vi "uart data_main — kopia.vi"() -> ()   [LabVIEW 2015]
uses:
  data_typedef.ctl
  C:/Users/Arkadiusz/SkyDrive/Dokumenty/NordicSemiconductor/LabVIEW/UART_Accelero/uart data_akcelerometr/NordicDatabaseDLL.dll
  NordicDatabaseDLL.dll
  <vilib>/Instr/_visa.llb/VISA Configure Serial Port (Instr).vi
panel:
  out "Accelero Chart":T1(graph)
  out "Temperature Chart":dbl[](graph)
  in  "stop":bool
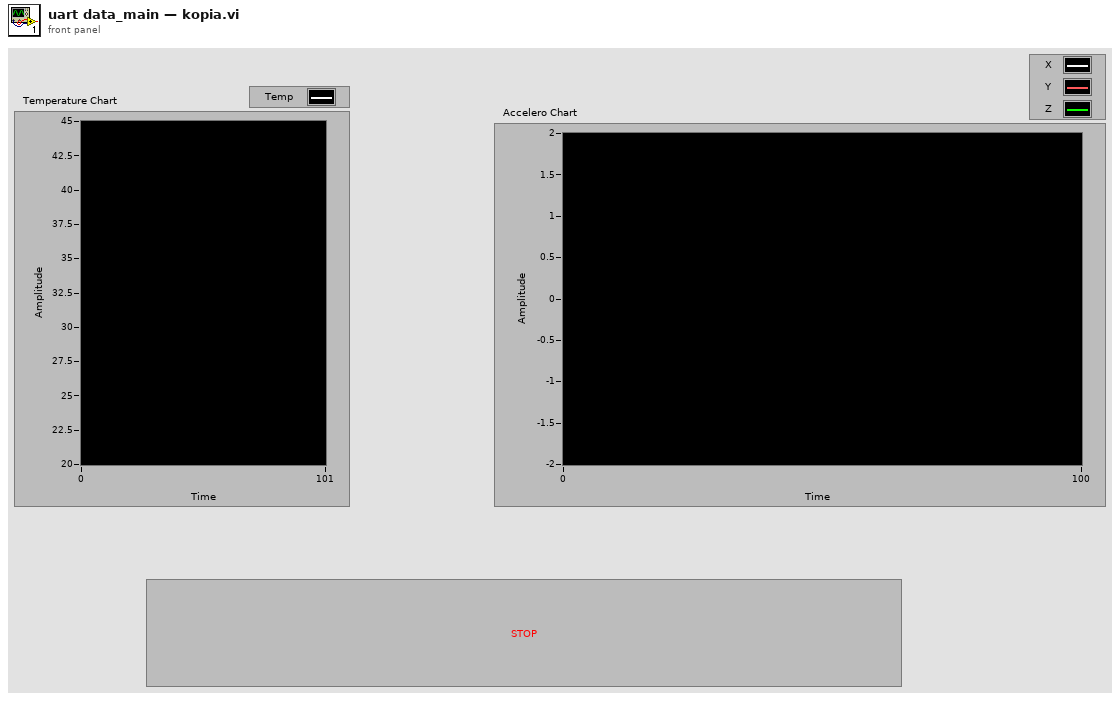
[diagram p1: front panel]
types:
  T1 = cluster{"X element out":dbl, "X element out":dbl, "Z element out":dbl}
  T2 = cluster{"Z element out":dbl, "X element out":dbl, "X element out 2":dbl}[]
  T3 = typedef "data_typedef.ctl" = cluster{"Accelero Array":dbl[], "Z out":dbl[], "Y out":dbl[], "X out":dbl[], "Numeric":i32}
  T4 = typedef "DBEnum.ctl" = enum16{"Temperature", "HeartRate", "XAccelero", "YAccelero", "ZAccelero"}
  T5 = cluster{"X element out":dbl, "Y element out":dbl, "Z element out":dbl}
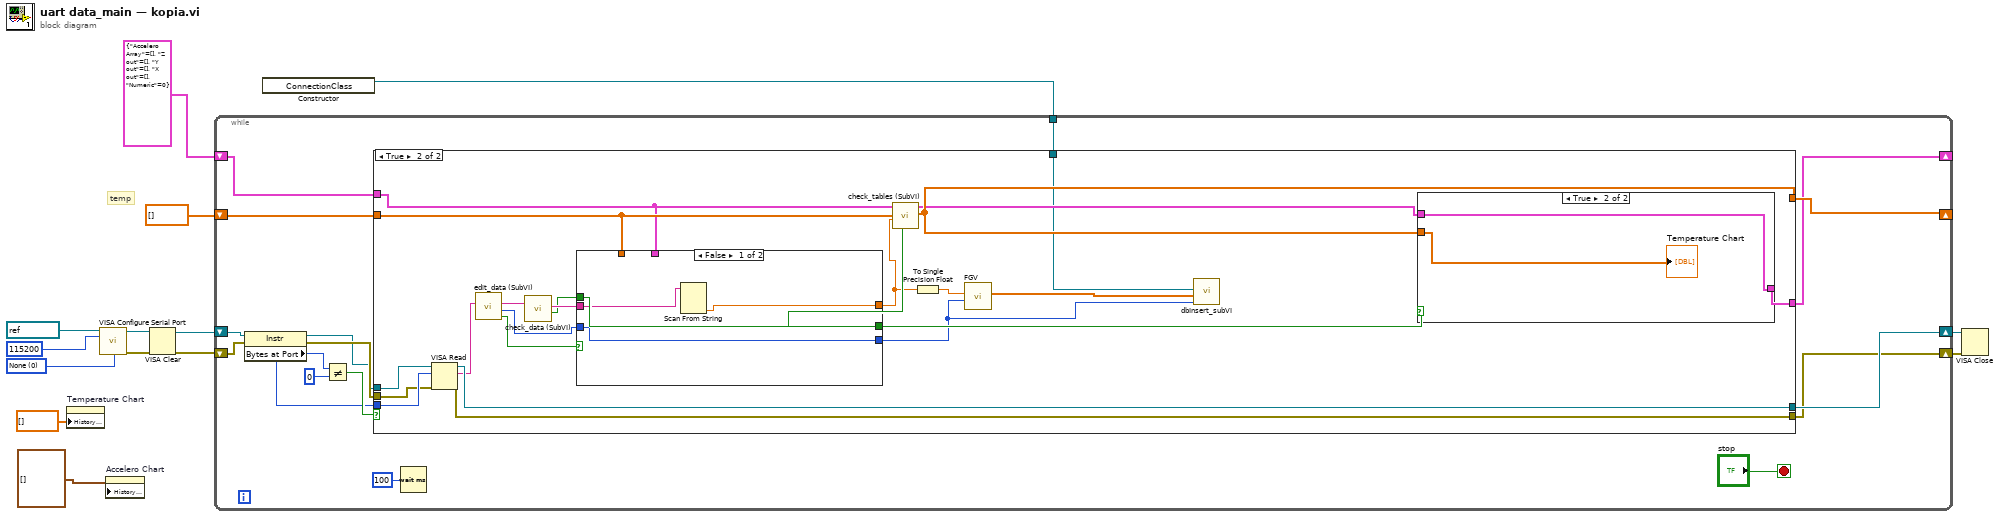
[diagram p0: block diagram]
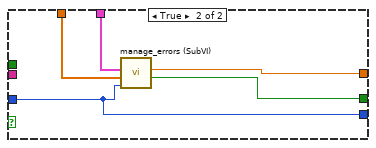
[diagram p3: hidden frame]
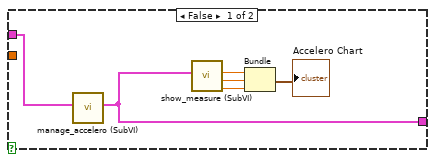
[diagram p4: hidden frame]
diagram:
  w10 = u16 0 items=["None", "XON/XOFF", "RTS/CTS", "XON/XOFF & RTS/CTS", "DTR/DSR", "XON/XOFF & DTR/DSR"] ("flow control (0:none)")
  # "temp"
  n1 = property on="Temperature Chart" class="WFChart (strict)"("History Data"=dbl[] []) -> ()  [unwired: 2 in, 2 out]
  n2 = call-poly "VISA Configure Serial Port"("VISA resource name"=refnum<visa-resource-name> "COM5", "baud rate (9600)"=u32 115200, "flow control (0:none)"=w10) -> ("VISA resource name out"=w6:refnum<visa-resource-name>, "error out"=w5:errorcluster)  [unwired: 11 in]
  n3 = property on="Accelero Chart" class="WFChart (strict)"("History Data"=T2 []) -> ()  [unwired: 2 in, 2 out]
  n4 = VISA Clear(VISA resource name=w6, error in (no error)=w5) -> (VISA resource name out=w7:refnum<visa-resource-name>, error out=w8:errorcluster)
  n5 = constructor class="ConnectionClass"() -> (reference out=w1:refnum<k24>)  [unwired: 3 in, 2 out]
  n6 = while {
    shift-right: [w29] -> w12
    shift-left: w7 -> [w28]
    shift-right: [w25] -> w11
    shift-left: w8 -> [w26]
    shift-right: [w18] -> _
    shift-left: dbl[] [] -> [w21]
    shift-right: [w16] -> _
    shift-left: T3 {"Accelero Array"=[], "Z out"=[], "Y out"=[], "X out"=[], "Numeric"=0} ("Tabs") -> [w17]
    tunnel: w1 -> [w15]
    stop <- "stop" stop-if-true
    # "main loop"
    n7 = property class="Instr"(reference=w28, error in=w26) -> (reference out=w24:refnum<visa-resource-name>, error out=w27:errorcluster, "Bytes at Port"=w20:u32)
    n8 = Not Equal?(x=w20, y=u32 0) -> (x != y?=w22:bool)
    n9 = case shown="True" w22 {
      tunnel: [w34 w56] -> w29
      tunnel: w20 -> [_ w55]
      tunnel: w27 -> [w33 w54]
      tunnel: [w33 w53] -> w25
      tunnel: w24 -> [w34 w52]
      tunnel: w21 -> [w32 w46]
      tunnel: [w32 w50] -> w18
      tunnel: w17 -> [w31 w44]
      tunnel: [w31 w49] -> w16
      tunnel: w15 -> [_ w36]
      frame False {
      }
      frame True {
        # "true"
        n10 = VISA Read(VISA resource name=w52, byte count=w55, error in (no error)=w54) -> (VISA resource name out=w56:refnum<visa-resource-name>, read buffer=w41:string, error out=w53:errorcluster)  [unwired: 1 out]
        n11 = call "edit_data (SubVI).vi"("data in"=w41) -> ("error bool out"=w42:bool, "Enum 2"=w43:T4, "data out"=w51:string)  [unwired: 8 in]
        n12 = call "check_data (SubVI).vi"("read buffer"=w51) -> ("buffer out"=w48:string, "bool out"=w47:bool)  [unwired: 8 in]
        n13 = case shown="False" w42 {
          tunnel: w48 -> [w59 _]
          tunnel: w47 -> [w60 _]
          tunnel: w46 -> [_ w64]
          tunnel: [w60 w65] -> w45
          tunnel: [w57 w61] -> w40
          tunnel: w43 -> [w58 w62]
          tunnel: w44 -> [_ w63]
          tunnel: [w58 w62] -> w35
          frame False {
            n14 = Scan From String(input string=w59) -> (output 1=w57:dbl)  [unwired: 4 in, 3 out]
          }
          frame True {
            n15 = call "manage_errors (SubVI).vi"("Enum"=w62, "Temperature Array"=w64, "Data in"=w63) -> ("Boolean out"=w65:bool, "Out value"=w61:dbl)  [unwired: 7 in]
          }
        }
        n16 = call "check_tables (SubVI).vi"("bool in"=w45, "numeric buffer in"=w40, "temperature array in"=w46, "Data in"=w44) -> ("temperature array out"=w50:dbl[], "Data out"=w39:T3)  [unwired: 6 in]
        n17 = To Single Precision Float(number=w40) -> (single precision float=w38:sgl)
        n18 = call "FGV.vi"("Enum"=w35, "Data in"=w38) -> ("Output Array"=w37:sgl[])  [unwired: 9 in]
        n19 = call "dbInsert_subVI.vi"("Enum"=w35, "Array"=w37, "reference"=w36) -> ()  [unwired: 9 in]
        n20 = case shown="True" w45 {
          tunnel: w50 -> [_ w73]
          tunnel: w39 -> [w67 w72]
          tunnel: [w66 w72] -> w49
          frame False {
            n21 = call "manage_accelero (SubVI).vi"("Data in"=w67) -> ("Data out"=w66:T3)  [unwired: 9 in]
            n22 = call "show_measure (SubVI).vi"("Data in"=w66) -> ("Z element out"=w70:dbl, "Y element out"=w68:dbl, "X element out"=w71:dbl)  [unwired: 8 in]
            n23 = Bundle("X element out"=w71, "Y element out"=w68, "Z element out"=w70) -> (→"Accelero Chart":T5)  [unwired: 1 in]
          }
          frame True {
            "Temperature Chart" <- w73
          }
        }
      }
    }
    n24 = Wait (ms)(milliseconds to wait=u32 100) -> ()  [unwired: 1 out]
  }
  n25 = VISA Close(VISA resource name=w12, error in (no error)=w11) -> ()  [unwired: 1 out]
